vi "SubpanelTemplate.vi"(11 "notifier":refnum<notifier>) -> ()   [LabVIEW 2013, in "main.lvlib"]
uses:
  main.lvlib
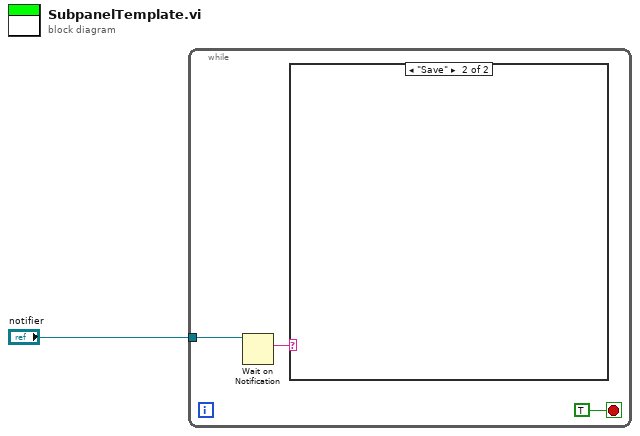
[diagram p0: block diagram]
diagram:
  n1 = while {
    tunnel: "notifier" -> [w3]
    stop <- TRUE stop-if-true
    n2 = Wait on Notification(notifier=w3) -> (notification=w4:string)  [unwired: 3 in, 3 out]
    n3 = case shown="\"Save\"" w4 {
      frame "Cancel", Default {
      }
      frame "Save" {
      }
    }
  }
